vi "Global scelta rpm.vi"() -> ()   [LabVIEW 2016]
panel:
  out "Rpm da fft?":bool
  out "Rpm tors":bool
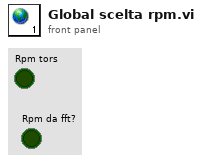
[diagram p1: front panel]
diagram:
